vi "test2.vi"() -> ()   [LabVIEW 2020]
panel:
  out "输出变量":i32
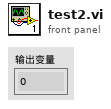
[diagram p1: front panel]
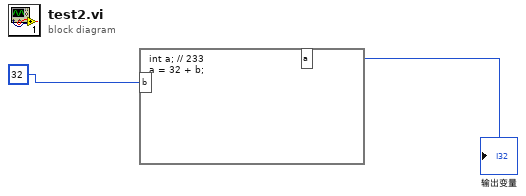
[diagram p0: block diagram]
diagram:
  n1 = formula code="int a; // 233\na = 32 + b;"("b"=32) -> ("a"=→"输出变量":i32)
